vi "destroy.vi"(8 "error in (no error)":errorcluster, 11 "DAQ View in":refnum<class "DAQ View.lvclass">) -> (0 "error out":errorcluster, 3 "DAQ View out":refnum<class "DAQ View.lvclass">)   [LabVIEW 2022 SP3, in "DAQ View.lvclass"]
uses:
  DAQ View.lvclass
  DAQ View.lvclass/DAQ View.ctl
  iView/base view/base view.lvclass
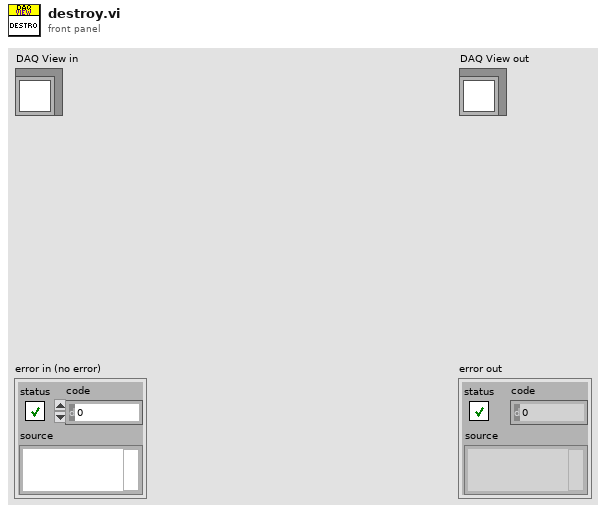
[diagram p1: front panel]
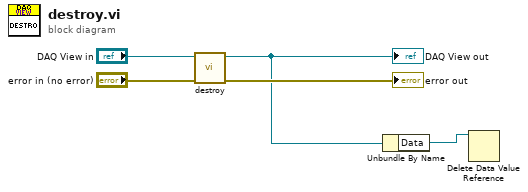
[diagram p0: block diagram]
diagram:
  n1 = call-parent "destroy.vi"("error in (no error)"="error in (no error)", "base view in"="DAQ View in") -> ("error out"=→"error out":errorcluster, "base view out"=w2:refnum<class "DAQ View.lvclass">)  [unwired: 8 in]
  "DAQ View out" <- w2
  n2 = Unbundle By Name(w2) -> ("Data"=w1:refnum<data-value>)
  n3 = Delete Data Value Reference(data value reference=w1) -> ()  [unwired: 1 in, 2 out]
